vi "Generate File Name.vi"() -> (2 "file name":string, 3 "system":string)   [LabVIEW 2020]
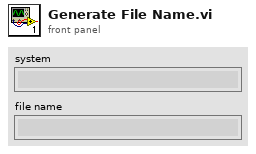
[diagram p1: front panel]
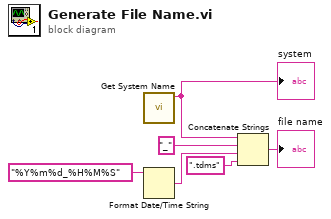
[diagram p0: block diagram]
diagram:
  n1 = call "Get System Name.vi"() -> ("name"=w2:string)  [unwired: 11 in]
  "system" <- w2
  n2 = Format Date/Time String(time format string (%c)="%Y%m%d_%H%M%S") -> (date/time string=w3:string)  [unwired: 2 in]
  n3 = Concatenate Strings(w2, "_" ("string"), w3, ".tdms" ("string")) -> (→"file name":string)
